vi "Queue Is Nested.vi"(10 "Alias":string, 11 "Base Event Actor in":refnum<class "Base Event Actor.lvclass">) -> (2 "Queue Is Nested?":bool)   [LabVIEW 2021, in "jettl.lvlib" / "Base Event Actor.lvclass"]
uses:
  Base Event Actor.lvclass
  Base Event Actor.lvclass/Base Event Actor.ctl
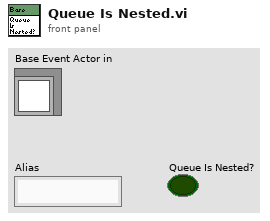
[diagram p1: front panel]
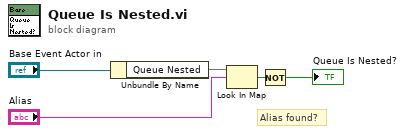
[diagram p0: block diagram]
diagram:
  # "Alias found?"
  n1 = Unbundle By Name("Base Event Actor in") -> ("Queue Nested"=w5:map{string, refnum<data-value>})
  n2 = Look In Map(map=w5, key="Alias") -> (key not found?=w4:bool)  [unwired: 1 in, 1 out]
  n3 = Not(x=w4) -> (.not. x?=→"Queue Is Nested?":bool)
